vi "Update.vi"(11 "Full App Name (ex: PC Interface.exe)":string="PC Interface.exe") -> ()   [LabVIEW 2019]
uses:
  controls/Update Cluster.ctl
  controls/Update Enum.ctl
panel:
  out "Error":string
  out "Title":string="Checking for PC Interface new version"
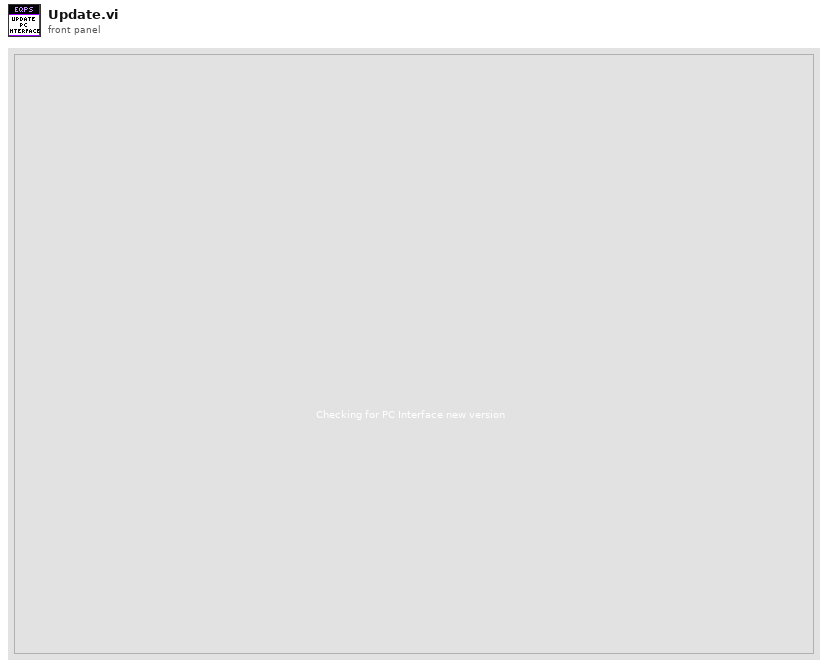
[diagram p1: front panel]
types:
  T1 = typedef "Update Cluster.ctl" = cluster{"Title":string, "Server Files Cluster":cluster{"aliases":string, "exe":string, "ini":string, "Server":path, "Version Array":i32[]}, "Local Version Array":i32[], "Temp path Array":path[], "Error Message":string}
  T2 = typedef "Update Enum.ctl" = enum16{"init", "read files", "check version", "kill app", "backup files", "delete files", "copy files", "recover files", "launching pc interface", "exit"}
  T3 = cluster{"aliases":string, "exe":string, "ini":string, "Server":path, "Version Array":i32[]}
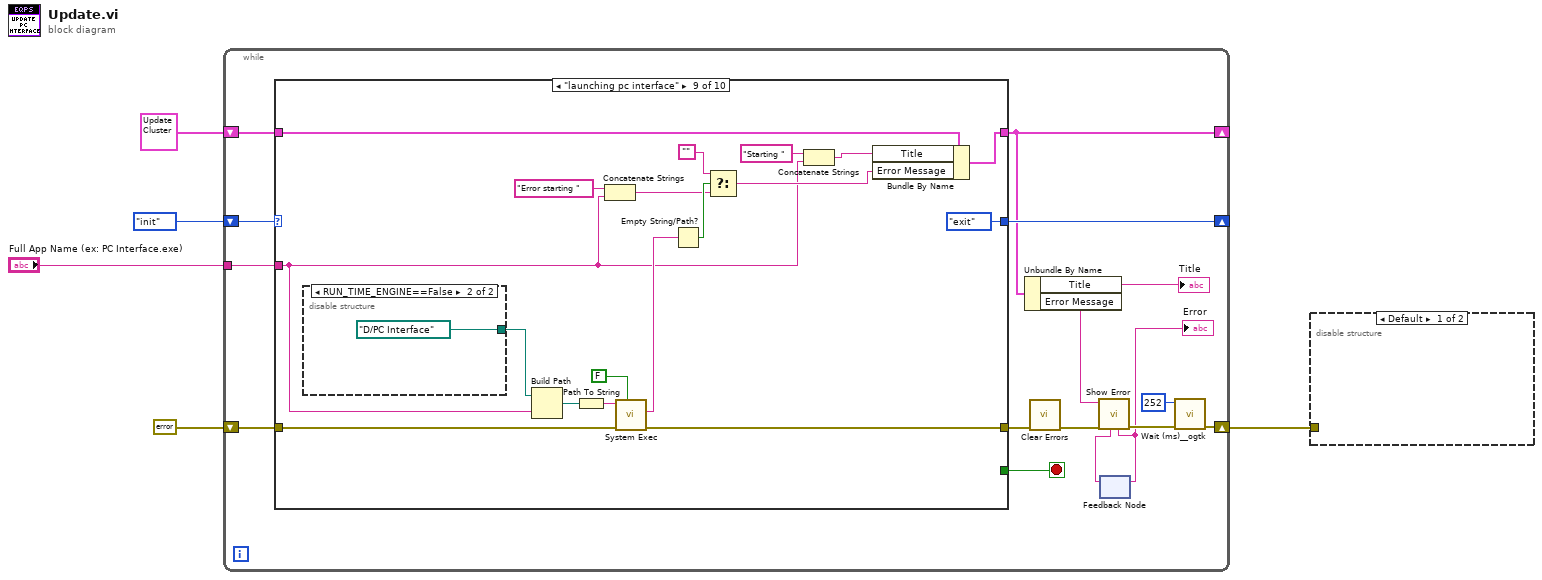
[diagram p0: block diagram]
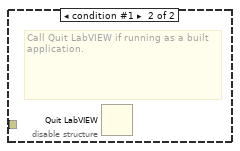
[diagram p2: hidden frame]
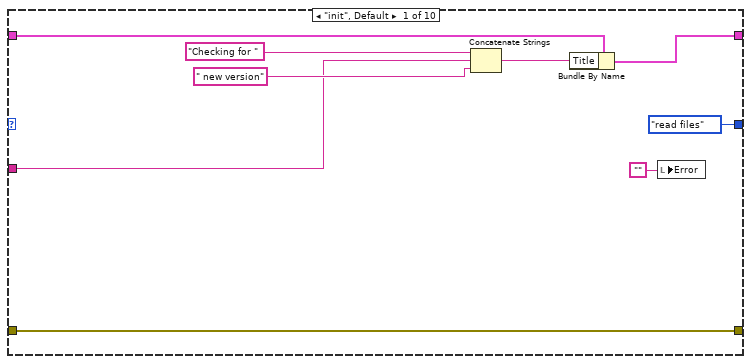
[diagram p3: hidden frame]
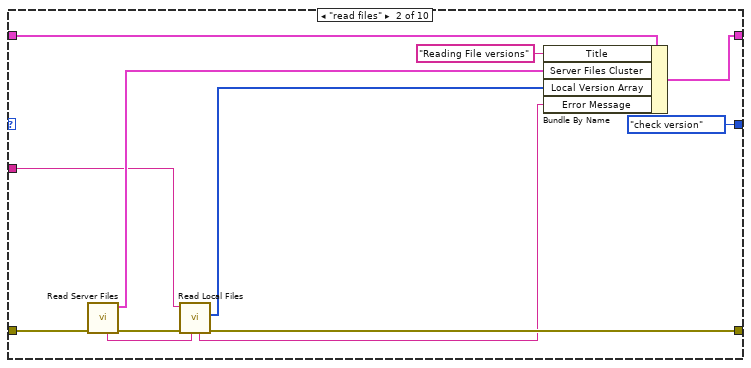
[diagram p4: hidden frame]
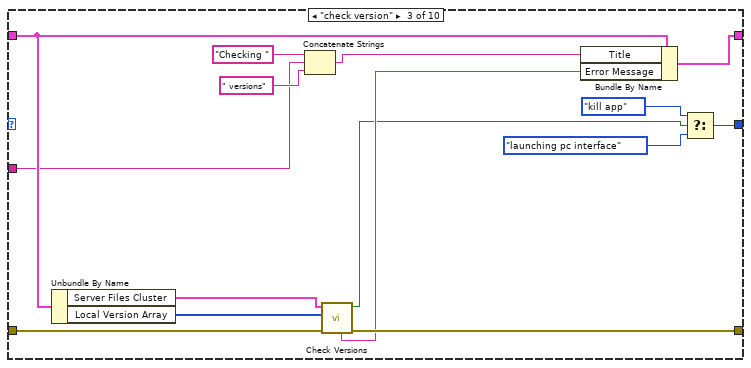
[diagram p5: hidden frame]
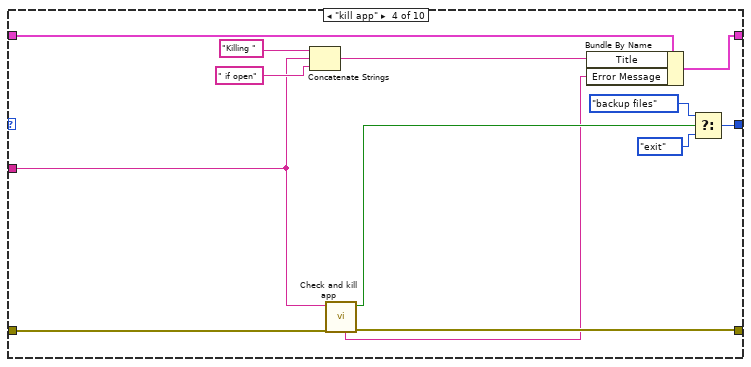
[diagram p6: hidden frame]
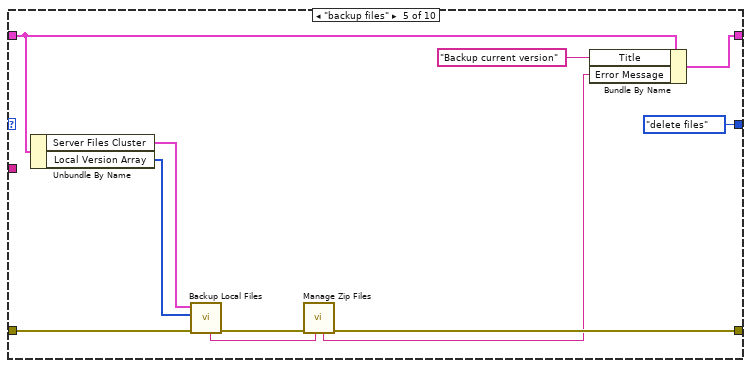
[diagram p7: hidden frame]
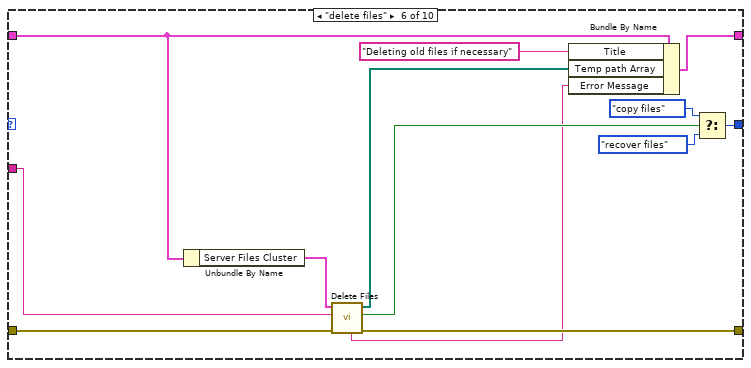
[diagram p8: hidden frame]
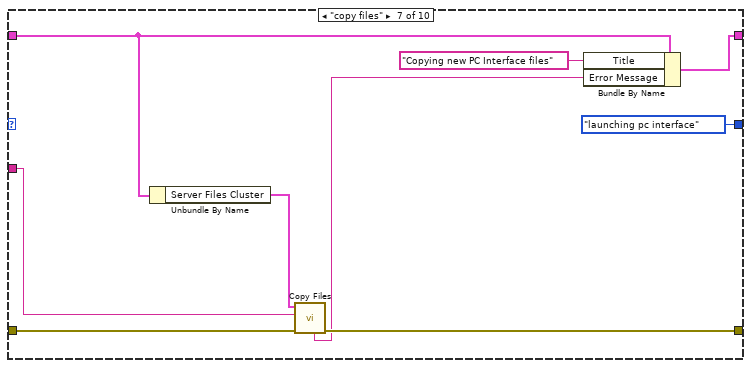
[diagram p9: hidden frame]
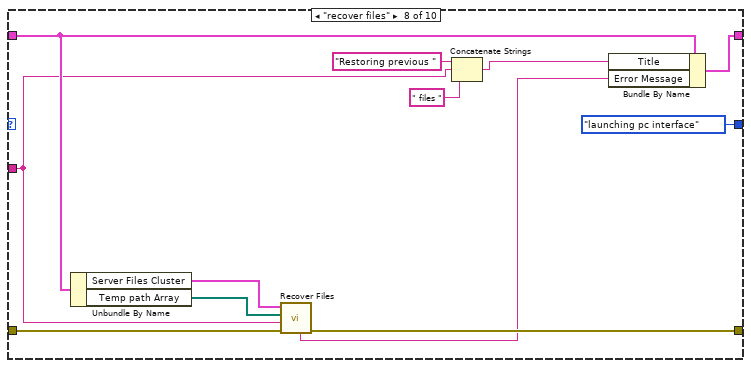
[diagram p10: hidden frame]
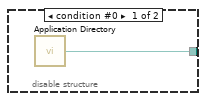
[diagram p11: hidden frame]
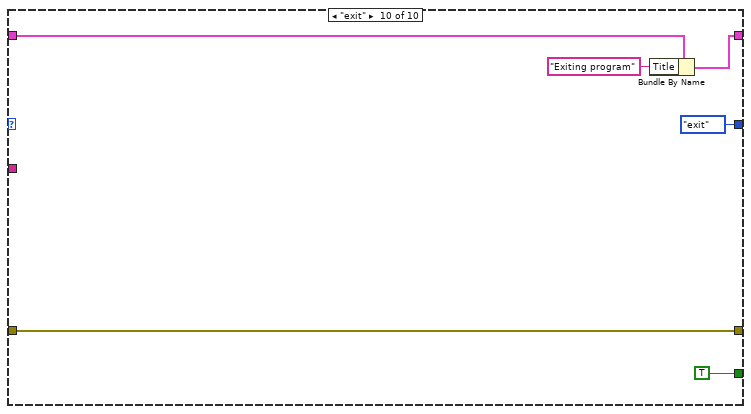
[diagram p12: hidden frame]
diagram:
  n1 = while {
    shift-right: [w20] -> _
    shift-left: Update_Enum."init" ("Update State") -> [w21]
    shift-right: [w8] -> w2
    shift-left: errorcluster {"status"=FALSE, "code"=0, "source"=""} ("error constant") -> [w18]
    shift-right: [w15] -> _
    shift-left: T1 {"Title"="", "Server Files Cluster"={"aliases"="", "exe"="", "ini"="", "Server"=path "", "Version Array"=[]}, "Local Version Array"=[], "Temp path Array"=[], "Error Message"=""} ("Update Cluster") -> [w16]
    tunnel: "Full App Name (ex: PC Interface.exe)" -> [w6]
    stop <- w19 stop-if-true
    n2 = case shown="\"launching pc interface\"" w21 {
      tunnel: [Update_Enum."read files" ("Update State") Update_Enum."check version" ("Update State") w51 w66 Update_Enum."delete files" ("Update State") w85 Update_Enum."launching pc interface" ("Update State") Update_Enum."launching pc interface" ("Update State") Update_Enum."exit" ("Update State") Update_Enum."exit" ("Update State")] -> w20
      tunnel: [_ _ _ _ _ _ _ _ _ TRUE] -> w19
      tunnel: w18 -> [w29 w41 w57 w70 w78 w94 w102 w114 w129 w139]
      tunnel: [w29 w35 w56 w69 w73 w93 w100 w111 w128 w139] -> w17
      tunnel: w16 -> [w28 w40 w50 w64 w77 w91 w99 w110 w133 w138]
      tunnel: [w27 w38 w49 w63 w80 w90 w98 w109 w132 w137] -> w15
      tunnel: w6 -> [w22 w31 w44 w58 _ w82 w95 w104 w116 _]
      frame "init", Default {
        n3 = Concatenate Strings("Checking for " ("Title"), w22, " new version" ("Title")) -> (w24:string)
        n4 = Bundle By Name(cluster=w28, "Title"=w24) -> (w27:T1)
        n5 = local write "Error"("") -> ()
      }
      frame "read files" {
        n6 = call "Read Server Files.vi"("Error In"=w41) -> ("Error Out"=w37:errorcluster, "Server Files Cluster"=w39:T3, "Error Message out"=w36:string)  [unwired: 8 in]
        n7 = call "Read Local Files.vi"("Error Message in"=w36, "Error In"=w37, "Full App Name"=w31) -> ("Error Out"=w35:errorcluster, "Local Version Array"=w34:i32[], "Error Message out"=w32:string)  [unwired: 6 in]
        n8 = Bundle By Name(cluster=w40, "Title"="Reading File versions", "Server Files Cluster"=w39, "Local Version Array"=w34, "Error Message"=w32) -> (w38:T1)
      }
      frame "check version" {
        n9 = Unbundle By Name(w50) -> ("Server Files Cluster"=w55:T3, "Local Version Array"=w54:i32[])
        n10 = Concatenate Strings("Checking " ("Title"), w44, " versions" ("Title")) -> (w46:string)
        n11 = call "Check Versions.vi"("Error In"=w57, "Local Version Array"=w54, "Server Files Cluster"=w55) -> ("Error Out"=w56:errorcluster, "Update Files"=w43:bool, "Error Message out"=w47:string)  [unwired: 6 in]
        n12 = Bundle By Name(cluster=w50, "Title"=w46, "Error Message"=w47) -> (w49:T1)
        n13 = Select(t=Update_Enum."kill app" ("Update State"), s=w43, f=Update_Enum."launching pc interface" ("Update State")) -> (s? t:f=w51:T2)
      }
      frame "kill app" {
        n14 = Concatenate Strings("Killing " ("Title"), w58, " if open" ("Title")) -> (w59:string)
        n15 = call "Check and kill app.vi"("Error In"=w70, "Full App name (ex: PC Interface.exe)"=w58) -> ("Error Out"=w69:errorcluster, "app closed"=w65:bool, "Error Message out"=w62:string)  [unwired: 7 in]
        n16 = Bundle By Name(cluster=w64, "Title"=w59, "Error Message"=w62) -> (w63:T1)
        n17 = Select(t=Update_Enum."backup files" ("Update State"), s=w65, f=Update_Enum."exit" ("Update State")) -> (s? t:f=w66:T2)
      }
      frame "backup files" {
        n18 = Unbundle By Name(w77) -> ("Server Files Cluster"=w76:T3, "Local Version Array"=w75:i32[])
        n19 = call "Backup Local Files.vi"("Error In"=w78, "Local Version Array"=w75, "Server Files Cluster"=w76) -> ("Error Out"=w74:errorcluster, "Error Message out"=w72:string)  [unwired: 7 in]
        n20 = call "Manage Zip Files.vi"("Error Message in"=w72, "Error In"=w74) -> ("Error Out"=w73:errorcluster, "Error Message out"=w71:string)  [unwired: 8 in]
        n21 = Bundle By Name(cluster=w77, "Title"="Backup current version", "Error Message"=w71) -> (w80:T1)
      }
      frame "delete files" {
        n22 = Unbundle By Name(w91) -> ("Server Files Cluster"=w92:T3)
        n23 = call "Delete Files.vi"("Error In"=w94, "Full App Name"=w82, "Server Files Cluster"=w92) -> ("Error Out"=w93:errorcluster, "Files Deleted"=w88:bool, "Temp path Array"=w89:path[], "Error Message out"=w83:string)  [unwired: 5 in]
        n24 = Bundle By Name(cluster=w91, "Title"="Deleting old files if necessary", "Temp path Array"=w89, "Error Message"=w83) -> (w90:T1)
        n25 = Select(t=Update_Enum."copy files" ("Update State"), s=w88, f=Update_Enum."recover files" ("Update State")) -> (s? t:f=w85:T2)
      }
      frame "copy files" {
        n26 = Unbundle By Name(w99) -> ("Server Files Cluster"=w101:T3)
        n27 = call "Copy Files.vi"("Error In"=w102, "Full App Name"=w95, "Server Files Cluster"=w101) -> ("Error Out"=w100:errorcluster, "Error Message out"=w96:string)  [unwired: 6 in, 1 out]
        n28 = Bundle By Name(cluster=w99, "Title"="Copying new PC Interface files", "Error Message"=w96) -> (w98:T1)
      }
      frame "recover files" {
        n29 = Unbundle By Name(w110) -> ("Server Files Cluster"=w113:T3, "Temp path Array"=w112:path[])
        n30 = call "Recover Files.vi"("Error In"=w114, "Full App Name"=w104, "Temp path Array"=w112, "Server Files Cluster"=w113) -> ("Error Out"=w111:errorcluster, "Error Message out"=w107:string)  [unwired: 5 in, 1 out]
        n31 = Concatenate Strings("Restoring previous " ("Title"), w104, " files " ("Title")) -> (w106:string)
        n32 = Bundle By Name(cluster=w110, "Title"=w106, "Error Message"=w107) -> (w109:T1)
      }
      frame "launching pc interface" {
        n33 = disable-structure shown="RUN_TIME_ENGINE==False" {
          disable-tunnel: [w134 path "D:/PC Interface"] -> w126
          frame condition #0 {
            n34 = call <vilib>:"Application Directory.vi"() -> ("Application Directory"=w134:path)
          }
          frame condition #1 (active) {
          }
        }
        n35 = Build Path(base path=w126, name or relative path=w116) -> (appended path=w125:path)
        n36 = Path To String(path=w125) -> (string=w124:string)
        n37 = Concatenate Strings("Error starting ", w116) -> (w118:string)
        n38 = call <vilib>:"System Exec.vi"("wait until completion? (T)"=FALSE, "error in (no error)"=w129, "command line"=w124) -> ("error out"=w128:errorcluster, "standard error"=w122:string)  [unwired: 5 in, 2 out]
        n39 = Empty String/Path?(string/path=w122) -> (empty?=w123:bool)
        n40 = Select(t="", s=w123, f=w118) -> (s? t:f=w119:string)
        n41 = Concatenate Strings("Starting " ("Title"), w116) -> (w117:string)
        n42 = Bundle By Name(cluster=w133, "Title"=w117, "Error Message"=w119) -> (w132:T1)
      }
      frame "exit" {
        n43 = Bundle By Name(cluster=w138, "Title"="Exiting program") -> (w137:T1)
      }
    }
    n44 = Unbundle By Name(w15) -> ("Title"=→"Title":string, "Error Message"=w10:string)
    n45 = call <vilib>:"Clear Errors.vi"("error in (no error)"=w17) -> ("error out"=w13:errorcluster)  [unwired: 5 in, 1 out]
    n46 = feedback #1() -> (w11:string)  [unwired: 1 in]
    n47 = call "Show Error.vi"("Last Error Message in"=w11, "Error In"=w13, "Error Message in"=w10) -> ("Error Out"=w12:errorcluster, "Error Message out"=w9:string)  [unwired: 7 in]
    "Error" <- w9
    n48 = feedback-in #1(w9) -> ()
    n49 = call <userlib>:"Wait (ms)__ogtk.vi"("error in (no error)"=w12, "milliseconds to wait"=u32 252) -> ("error out"=w8:errorcluster)  [unwired: 8 in, 1 out]
  }
  n50 = disable-structure shown="Default" {
    disable-tunnel: w2 -> [_ _]
    frame condition #0 (active) {
    }
    frame condition #1 {
      # "Call Quit LabVIEW if running as a built application."
      n51 = Quit LabVIEW() -> ()  [unwired: 1 in]
    }
  }
